vi "Move FP and BD.vi"() -> ()   [LabVIEW 2013]
panel:
  in  "contains dialogs":bool
  out "error out":errorcluster
  in  "Path":path=path "C:/"
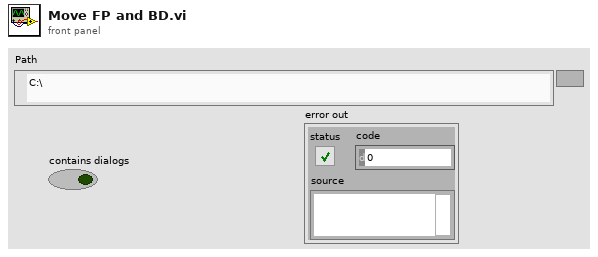
[diagram p1: front panel]
types:
  T1 = typedef "LVRectTypeDef.ctl" = cluster{"Left":i16, "Top":i16, "Right":i16, "Bottom":i16}
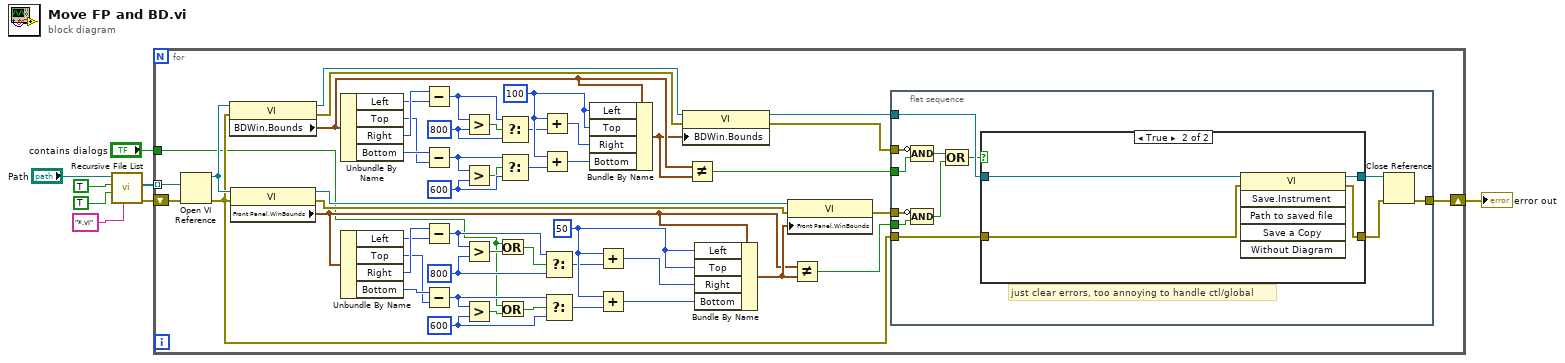
[diagram p0: block diagram]
diagram:
  n1 = call <vilib>:"Recursive File List.vi"("pattern"="*.vi", "Continue Recursing on Error? (F)"=TRUE, "Treat LLBs as Folders?"=TRUE, "Folder Path"="Path") -> ("error out"=w4:errorcluster, "All Files in Dir"=w3:path[])  [unwired: 3 in, 3 out]
  n2 = for {
    shift-right: [w57] -> w2
    shift-left: w4 -> [w59]
    tunnel: w3 -> [w58] mode=indexing
    tunnel: "contains dialogs" -> [w9]
    w44 = i16 600 ("y")
    w43 = i16 800 ("y")
    w49 = i16 600 ("y")
    w50 = i16 800 ("y")
    w33 = i16 50 ("Left")
    w34 = i16 100 ("Left")
    n3 = Open VI Reference(vi path=w58, error in (no error)=w59) -> (vi reference=w22:refnum<vi>, error out=w14:errorcluster)  [unwired: 4 in]
    n4 = property class="VI"(reference=w22, error in=w14) -> (reference out=w55:refnum<vi>, error out=w56:errorcluster, "BDWin.Bounds"=w18:T1)
    n5 = property class="VI"(reference=w22, error in=w14) -> (reference out=w23:refnum<vi>, error out=w21:errorcluster, "Front Panel.WinBounds"=w15:T1)
    n6 = Unbundle By Name(w18) -> ("Left"=w53:i16, "Top"=w37:i16, "Right"=w54:i16, "Bottom"=w38:i16)
    n7 = Unbundle By Name(w15) -> ("Left"=w39:i16, "Top"=w35:i16, "Right"=w40:i16, "Bottom"=w36:i16)
    n8 = Subtract(x=w54, y=w53) -> (x-y=w51:i16)
    n9 = Subtract(x=w38, y=w37) -> (x-y=w48:i16)
    n10 = Subtract(x=w40, y=w39) -> (x-y=w42:i16)
    n11 = Subtract(x=w36, y=w35) -> (x-y=w45:i16)
    n12 = Greater?(x=w51, y=w50) -> (0:w52:bool)
    n13 = Greater?(x=w48, y=w49) -> (0:w47:bool)
    n14 = Greater?(x=w42, y=w43) -> (0:w41:bool)
    n15 = Greater?(x=w45, y=w44) -> (0:w46:bool)
    n16 = Or(x=w9, y=w41) -> (x .or. y?=w11:bool)
    n17 = Or(x=w9, y=w46) -> (x .or. y?=w10:bool)
    n18 = Select(t=w51, s=w52, f=w50) -> (s? t:f=w29:i16)
    n19 = Select(t=w48, s=w47, f=w49) -> (s? t:f=w30:i16)
    n20 = Add(x=w34, y=w29) -> (x+y=w28:i16)
    n21 = Add(x=w34, y=w30) -> (x+y=w27:i16)
    n22 = Select(t=w42, s=w11, f=w43) -> (s? t:f=w32:i16)
    n23 = Select(t=w45, s=w10, f=w44) -> (s? t:f=w31:i16)
    n24 = Bundle By Name(cluster=w18, "Left"=w34, "Top"=w34, "Right"=w28, "Bottom"=w27) -> (w17:T1)
    n25 = Add(x=w33, y=w32) -> (x+y=w26:i16)
    n26 = Add(x=w33, y=w31) -> (x+y=w25:i16)
    n27 = property class="VI"(reference=w55, error in=w56, "BDWin.Bounds"=w17) -> (reference out=w24:refnum<vi>, error out=w20:errorcluster)
    n28 = Not Equal?(x=w18, y=w17) -> (x != y?=w13:bool)
    n29 = Bundle By Name(cluster=w15, "Left"=w33, "Top"=w33, "Right"=w26, "Bottom"=w25) -> (w16:T1)
    n30 = property class="VI"(reference=w23, error in=w21, "Front Panel.WinBounds"=w16) -> (error out=w19:errorcluster)  [unwired: 1 out]
    n31 = Not Equal?(x=w15, y=w16) -> (x != y?=w12:bool)
    n32 = flat-sequence {
      tunnel: [w71] -> w57
      tunnel: w24 -> [w70]
      tunnel: w20 -> [w66]
      tunnel: w19 -> [w64]
      tunnel: w14 -> [w67]
      tunnel: w13 -> [w65]
      tunnel: w12 -> [w63]
      frame #0 {
        # "just clear errors, too annoying to handle ctl/global"
        n33 = Compound Arithmetic op=AND(invert w66, w65) -> (w61:bool)
        n34 = Compound Arithmetic op=AND(invert w64, w63) -> (w60:bool)
        n35 = Compound Arithmetic op=OR(w61, w60) -> (w62:bool)
        n36 = case shown="True" w62 {
          tunnel: w70 -> [w73 w77]
          tunnel: [w72 w76] -> w69
          tunnel: [w73 w75] -> w68
          tunnel: w67 -> [w72 w74]
          frame False {
          }
          frame True {
            n37 = invoke class="VI" method="Save.Instrument"(reference=w77, error in=w74) -> (reference out=w75:refnum<vi>, error out=w76:errorcluster)  [unwired: 4 in, 4 out]
          }
        }
        n38 = Close Reference(reference=w68, error in (no error)=w69) -> (error out=w71:errorcluster)
      }
    }
  }
  "error out" <- w2
